vi "Swerve Sanity Check.vi"(4 "Current Pod Setpoints":dbl[](array[numeric]), 5 "Throttle In":dbl[](array[numeric]), 7 "Steer In":dbl[](array[numeric])) -> (1 "Throttle Out":dbl[](array[numeric]), 3 "Steer Out":dbl[](array[numeric]))   [LabVIEW 2020]
uses:
  <vilib>/Analysis/coordinate.llb/Angle Units.ctl
  <vilib>/Analysis/coordinate.llb/Absolute Angle Difference (array).vi
  <vilib>/Analysis/coordinate.llb/Wrap Angle (array).vi
  <vilib>/Analysis/coordinate.llb/Set Angle Unit.vi
  <vilib>/Analysis/NI_AAL_Angle.lvlib
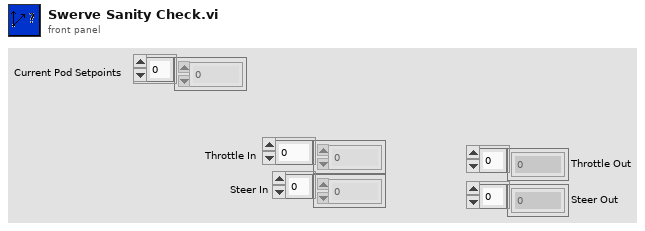
[diagram p1: front panel]
types:
  T1 = typedef "NI_AAL_Angle.lvlib/Angle Units.ctl" = i32
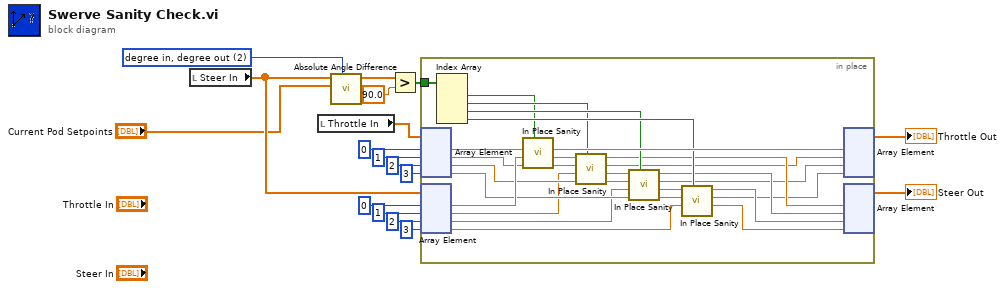
[diagram p0: block diagram]
diagram:
  w16 = T1 2 items=["radian in, radian out", "radian in, degree out", "degree in, degree out", "degree in, radian out"] ("angle units")
  n1 = local read "Steer In"() -> (w15:dbl[])
  n2 = local read "Throttle In"() -> (w17:dbl[])
  n3 = call-poly <vilib>:"Absolute Angle Difference.vi"("angle units"=w16, "Angle 2"="Current Pod Setpoints", "Angle 1"=w15) -> ("Absolute Angle Difference"=w13:dbl[])  [unwired: 7 in, 1 out]
  n4 = Greater?(x=w13, y=90.0) -> (0:w12:bool[])
  n5 = in-place {
    in-place-border: w12 -> [w29]
    n6 = in-place-array #1(w17, 0, 1, 2, 3) -> (w37:dbl, w36:dbl, w35:dbl, w34:dbl)
    n7 = in-place-array #2(w15, 0, 1, 2, 3) -> (w38:dbl, w33:dbl, w32:dbl, w31:dbl)
    n8 = Index Array(array=w29) -> (element #1=w25:bool, element #2=w26:bool, element #3=w27:bool, element #4=w28:bool)  [unwired: 4 in]
    n9 = call "In Place Sanity.vi"("Reversed?"=w25, "Steer In"=w38, "Throttle In"=w37) -> ("Steer Out"=w24:dbl, "Throttle Out"=w30:dbl)  [unwired: 5 in]
    n10 = call "In Place Sanity.vi"("Reversed?"=w26, "Steer In"=w33, "Throttle In"=w36) -> ("Steer Out"=w22:dbl, "Throttle Out"=w23:dbl)  [unwired: 5 in]
    n11 = call "In Place Sanity.vi"("Reversed?"=w27, "Steer In"=w32, "Throttle In"=w35) -> ("Steer Out"=w20:dbl, "Throttle Out"=w21:dbl)  [unwired: 5 in]
    n12 = call "In Place Sanity.vi"("Reversed?"=w28, "Steer In"=w31, "Throttle In"=w34) -> ("Steer Out"=w18:dbl, "Throttle Out"=w19:dbl)  [unwired: 5 in]
    n13 = in-place-array #1(w30, w23, w21, w19) -> (→"Throttle Out":dbl[])  [unwired: 4 out]
    n14 = in-place-array #2(w24, w22, w20, w18) -> (→"Steer Out":dbl[])  [unwired: 4 out]
  }
